vi "wf_multi_master.vi"(4 "lower limit":dbl=2.0, 5 "template":string="SOUR<channel>:VOLT <value>;", 6 "upper limit":dbl format="%#_13g", 7 "format":string="%g", 8 "error in (no error)":errorcluster, 9 "options (rescale)":string, 10 "value":dbl) -> (0 "error out":errorcluster, 2 "value out":dbl=0.3)   [LabVIEW 2017]
uses:
  <vilib>/Instr/_visa.llb/Select Event Type.ctl
  hardware/serial/serial.lvlib
panel:
  out "ch1/ ch2 rescale (set with option, e.g: 1.0, 0.5)":dbl[](array[numeric])=[1.0, 0.5]
  in  "VISA":refnum<visa-resource-name>[](array[refnum])=["waveform_gen", "GPIB0::11::INSTR"]
  out "cmds":string="SOUR1:VOLT 0.300000;\r\nSOUR2:VOLT 0.150000;"
  in  "send":bool=TRUE
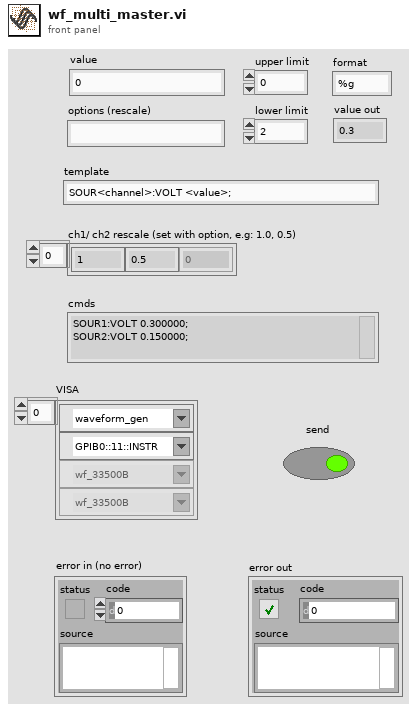
[diagram p1: front panel]
types:
  T1 = typedef "Select Event Type.ctl" = u32
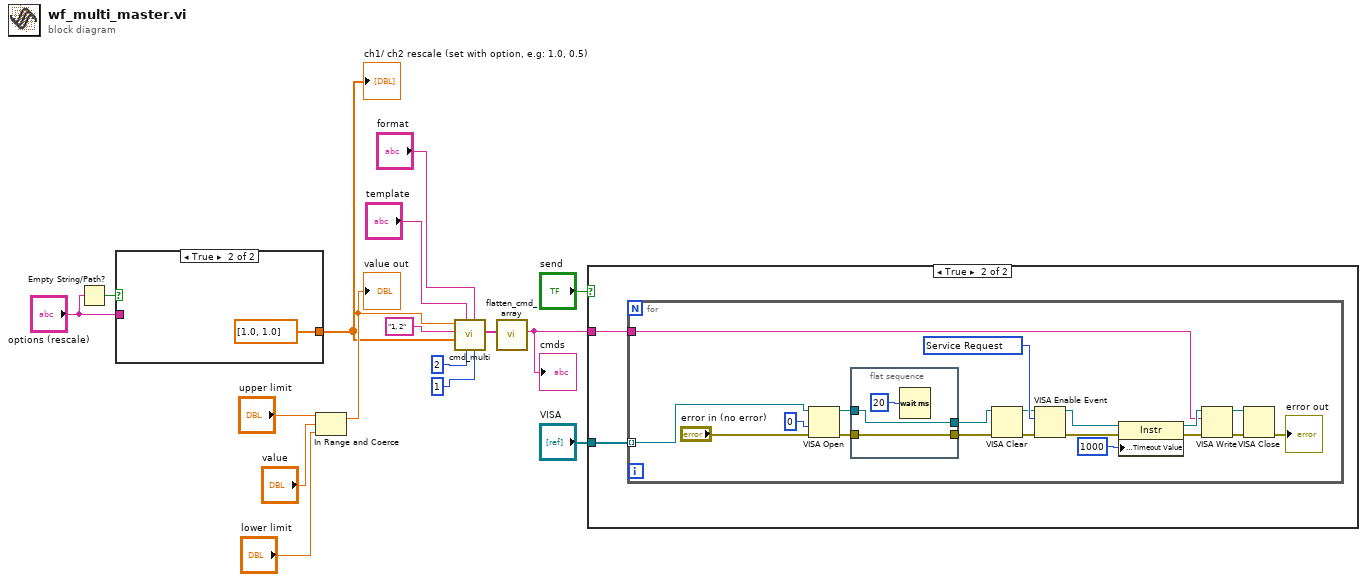
[diagram p0: block diagram]
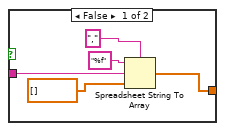
[diagram p2: hidden frame]
diagram:
  n1 = Empty String/Path?(string/path="options (rescale)") -> (empty?=w4:bool)
  n2 = case shown="True" w4 {
    tunnel: "options (rescale)" -> [w18 _]
    tunnel: [w17 dbl[] [1.0, 1.0]] -> w3
    frame False {
      n3 = Spreadsheet String To Array(delimiter (Tab)=",", format string="%f", spreadsheet string=w18, array type (2D Dbl)=dbl[] []) -> (array=w17:dbl[])
    }
    frame True {
    }
  }
  "ch1/ ch2 rescale (set with option, e.g: 1.0, 0.5)" <- w3
  n4 = In Range and Coerce(upper limit="upper limit", x="value", lower limit="lower limit") -> (coerced(x)=w11:dbl)  [unwired: 1 out]
  "value out" <- w11
  n5 = call "cmd_multi.vi"("chan_lower limit"=1, "value format"="format", "chan_upper limit"=2, "template"="template", "scale_channels"=w3, "channel_list"="1, 2", "value"=w11) -> ("cmds"=w8:string[])  [unwired: 3 in, 1 out]
  n6 = call "flatten_cmd_array.vi"("cmd_array"=w8) -> ("cmds"=w7:string)  [unwired: 10 in]
  "cmds" <- w7
  n7 = case shown="True" "send" {
    tunnel: w7 -> [_ w24]
    tunnel: "VISA" -> [_ w23]
    frame False {
    }
    frame True {
      n8 = for {
        tunnel: w24 -> [w26]
        tunnel: w23 -> [w25] mode=indexing
        w34 = T1 1073684491 items=["Service Request"=1073684491, "Trigger"=3221168138, "Clear"=1073684493, "VXI Signal"=1073684512, "VXI/VME Interrupt"=3221168161, "VXI/VME Sysfail"=1073684509, "VXI/VME Sysreset"=1073684510, "GPIB CIC"=1073684498, "GPIB Talk"=1073684499, "GPIB Listen"=1073684500, "PXI Interrupt"=1073684514, "Serial Break"=1073684515, "Serial TermChar"=1073684516, "Serial CTS"=1073684521, "Serial DSR"=1073684522, "Serial DCD"=1073684524, "Serial RI"=1073684526, "Serial Character"=1073684533, "USB Interrupt"=1073684535, "All Enabled"=1073709055] ("Event Type")
        n9 = VISA Open(access mode=u32 0, error in (no error)="error in (no error)", VISA resource name=w25) -> (VISA resource name=w36:refnum<visa-resource-name>, error out=w38:errorcluster)  [unwired: 2 out]
        n10 = flat-sequence {
          tunnel: w38 -> [w46]
          tunnel: [w46] -> w37
          tunnel: w36 -> [w45]
          tunnel: [w45] -> w35
          frame #0 {
            n11 = Wait (ms)(milliseconds to wait=u32 20) -> ()  [unwired: 1 out]
          }
        }
        n12 = VISA Clear(VISA resource name=w35, error in (no error)=w37) -> (VISA resource name out=w33:refnum<visa-resource-name>, error out=w32:errorcluster)
        n13 = VISA Enable Event(8:w32, 10:w34, 11:w33) -> (0:w31:errorcluster, 3:w30:refnum<visa-resource-name>)  [unwired: 1 in]
        n14 = property class="Instr"(reference=w30, error in=w31, "General Settings:Timeout Value"=u32 1000) -> (reference out=w29:refnum<visa-resource-name>, error out=w39:errorcluster)
        n15 = VISA Write(VISA resource name=w29, write buffer=w26, error in (no error)=w39) -> (VISA resource name out=w27:refnum<visa-resource-name>, error out=w28:errorcluster)  [unwired: 1 out]
        n16 = VISA Close(VISA resource name=w27, error in (no error)=w28) -> (error out=→"error out":errorcluster)
      }
    }
  }
